vi "完整帧.vi"(3 "不完整帧":u8[](array[numeric]) format="%.0x") -> (1 "完整帧":u8[](array[numeric]) format="%.0x")   [LabVIEW 2014]
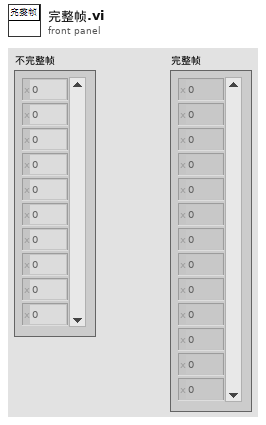
[diagram p1: front panel]
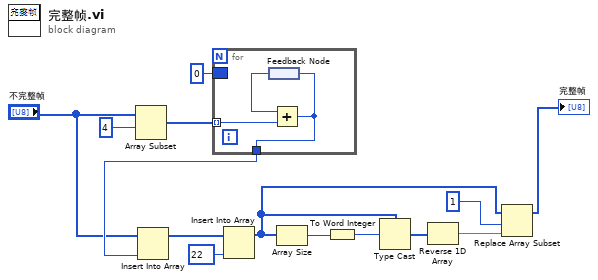
[diagram p0: block diagram]
diagram:
  n1 = Array Subset(array="不完整帧", index=4 ("长度")) -> (w8:u8[])  [unwired: 1 in]
  n2 = for {
    tunnel: w8 -> [w17] mode=indexing
    border: u8 0 -> [_]
    tunnel: [w15] -> w12
    n3 = feedback #1() -> (w16:u8)
    n4 = Add(x=w16, y=w17) -> (x+y=w15:u8)
    n5 = feedback-in #1(w15) -> ()
  }
  n6 = Insert Into Array(array="不完整帧", new element=w12) -> (w11:u8[])  [unwired: 1 in]
  n7 = Insert Into Array(array=w11, new element=u8 22 ("新元素/子数组")) -> (w3:u8[])  [unwired: 1 in]
  n8 = Array Size(array=w3) -> (size(s)=w9:i32)
  n9 = To Word Integer(number=w9) -> (16bit integer=w4:i16)
  n10 = Type Cast(type=w3, x=w4) -> (*(type *) &x=w7:u8[])
  n11 = Reverse 1D Array(array=w7) -> (reversed array=w6:u8[])
  n12 = Replace Array Subset(array=w3, new element=w6, index=1 ("索引")) -> (→"完整帧":u8[])
